vi "E6_Arrays.vi"() -> ()   [LabVIEW 2020]
panel:
  out "subarray 2":i32[](array[numeric])
  out "size(s) 2":i32
  out "size(s)":i32
  out "appended array":i32[][](array[numeric])
  out "element 8":dbl
  out "element 7":u16
  out "element 6":string
  out "element 5":bool
  in  "Array 4":dbl[][](array[numeric])
  in  "Array 3":u16[](array[numeric])
  in  "Array 2":string[](array[string])
  in  "Array":bool[](array[boolean])
  out "element 4":i32
  out "subarray":i32[](array[numeric])
  out "element 3":bool
  out "element 2":string
  out "element":dbl
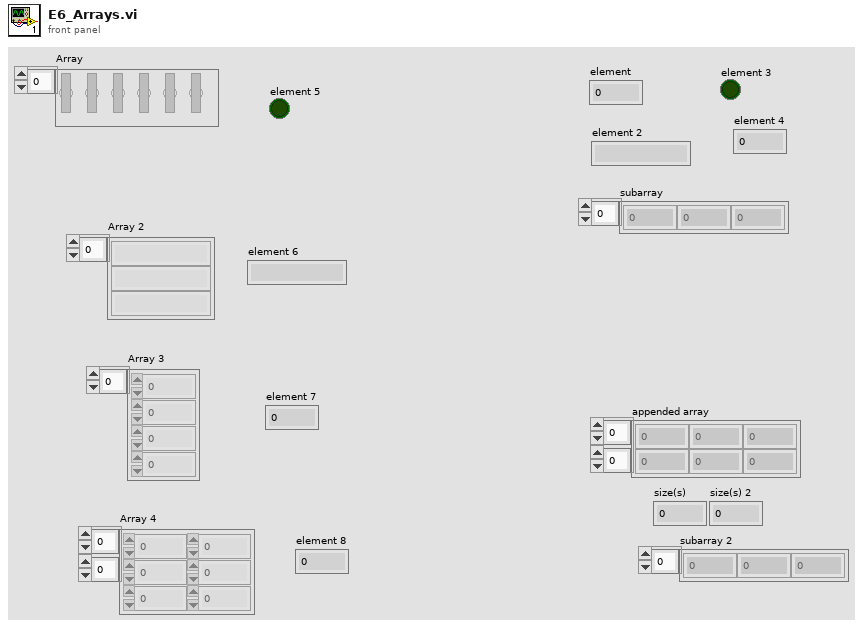
[diagram p1: front panel]
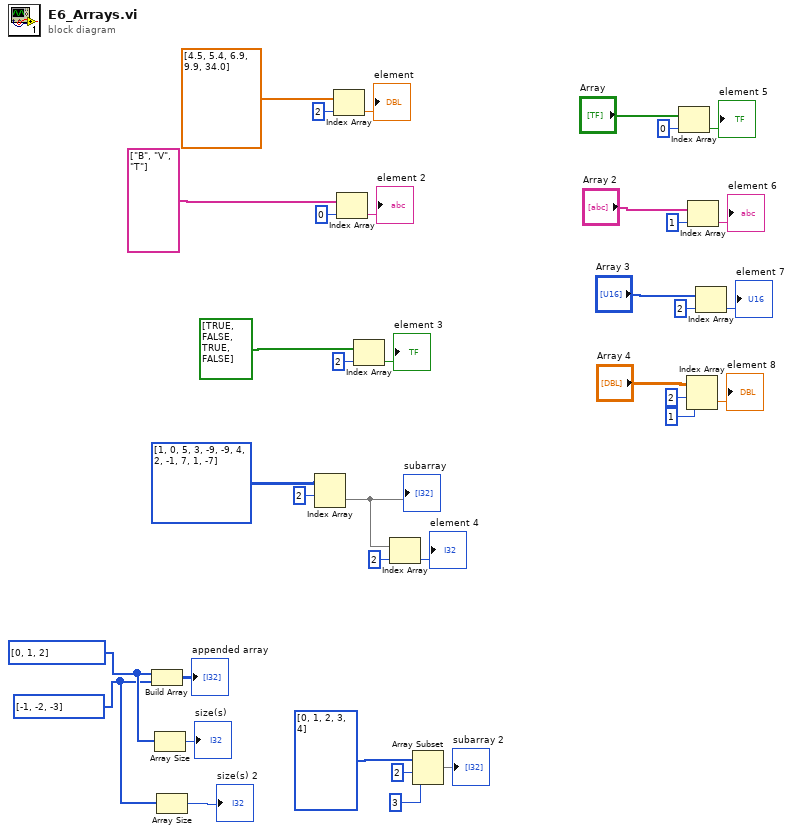
[diagram p0: block diagram]
diagram:
  w7 = i32[] [-1, -2, -3]
  w8 = i32[] [0, 1, 2]
  n1 = Build Array(w8, w7) -> (→"appended array":i32[][])
  n2 = Array Size(array=w8) -> (size(s)=→"size(s)":i32)
  n3 = Array Size(array=w7) -> (size(s)=→"size(s) 2":i32)
  n4 = Index Array(array=i32[][] [[1, 0, 5], [3, -9, -9], [4, 2, -1], [7, 1, -7]], index (row)=2) -> (element=w25:i32[])  [unwired: 1 in]
  "subarray" <- w25
  n5 = Index Array(array=dbl[] [4.5, 5.4, 6.9, 9.9, 34.0], index=2) -> (element=→"element":dbl)
  n6 = Index Array(array=string[] ["B", "V", "T"], index=0) -> (element=→"element 2":string)
  n7 = Index Array(array=bool[] [TRUE, FALSE, TRUE, FALSE], index=2) -> (element=→"element 3":bool)
  n8 = Index Array(array=w25, index=2) -> (element=→"element 4":i32)
  n9 = Array Subset(array=i32[] [0, 1, 2, 3, 4], index=2, length=3) -> (→"subarray 2":i32[])
  n10 = Index Array(array="Array", index=0) -> (element=→"element 5":bool)
  n11 = Index Array(array="Array 4", index (row)=2, index (col)=1 ("disabled index (col)")) -> (element=→"element 8":dbl)
  n12 = Index Array(array="Array 2", index=1) -> (element=→"element 6":string)
  n13 = Index Array(array="Array 3", index=2) -> (element=→"element 7":u16)
